vi "console.vi"() -> ()   [LabVIEW 2015]
uses:
  C:/Users/Giuseppe/Downloads/LabLinda_ pakage/index_datatype.ctl
  C:/Users/Giuseppe/Downloads/LabLinda_ pakage/index_cluster.ctl
panel:
  out "Array":cluster{i32}[](array[cluster])
  out "OUTVI REF":string[](array[string])
  out "Key_index":string[](array[string])
  out "Inited ?":bool
  out "IN VI Ref":string[](array[string])
  out "main index":i32
  in  "stop":bool
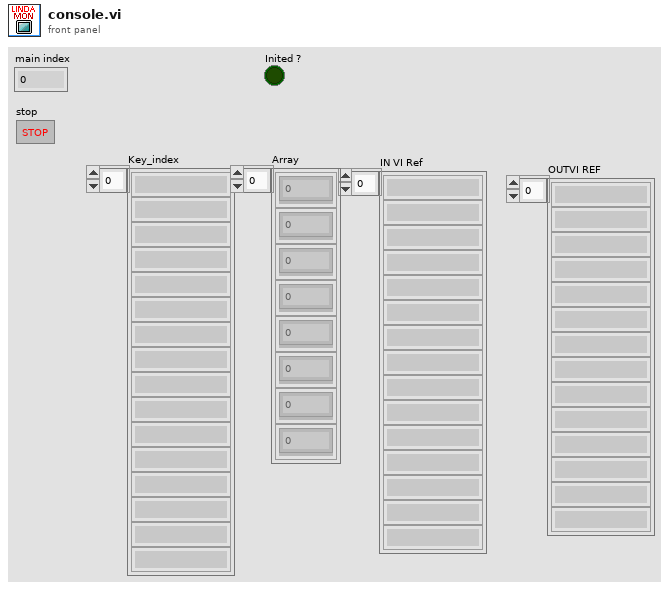
[diagram p1: front panel]
types:
  T1 = typedef "index_datatype.ctl" = T2[]
  T2 = typedef "index_cluster.ctl" = cluster{"Addr":i32[], "out react vi reference":refnum<vi>, "in react vi reference":refnum<vi>, "rd react vi reference":refnum<vi>, "Read_write_var":refnum<vi>}
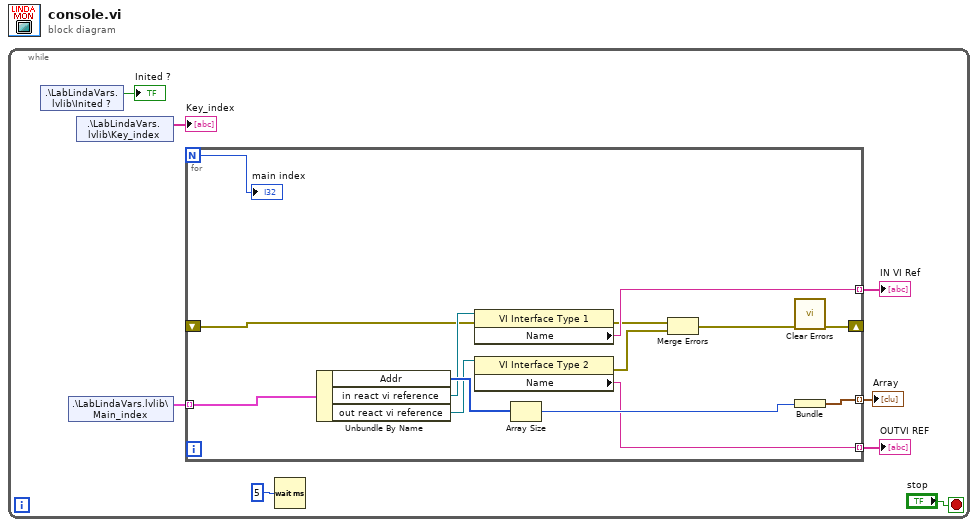
[diagram p0: block diagram]
diagram:
  n1 = while {
    stop <- "stop" stop-if-true
    n2 = shared-variable ".\\LabLindaVars.lvlib\\Inited ?"() -> (→"Inited ?":bool)  [unwired: 1 in, 1 out]
    n3 = shared-variable ".\\LabLindaVars.lvlib\\Main_index"() -> (w5:T1)  [unwired: 1 in, 1 out]
    n4 = shared-variable ".\\LabLindaVars.lvlib\\Key_index"() -> (→"Key_index":string[])  [unwired: 1 in, 1 out]
    n5 = for {
      N -> [w18]
      tunnel: w5 -> [w22] mode=indexing
      tunnel: [w19] -> w1 mode=indexing
      tunnel: [w16] -> w4 mode=indexing
      shift-right: [w14] -> _
      shift-left: _ -> [w15]
      tunnel: [w10] -> w2 mode=indexing
      n6 = Unbundle By Name(w22) -> ("Addr"=w21:i32[], "in react vi reference"=w17:refnum<vi>, "out react vi reference"=w13:refnum<vi>)
      n7 = property class="VI Interface Type 1"(reference=w17, error in=w15) -> (error out=w12:errorcluster, "Name"=w16:string)  [unwired: 1 out]
      n8 = property class="VI Interface Type 2"(reference=w13) -> (error out=w9:errorcluster, "Name"=w10:string)  [unwired: 1 in, 1 out]
      n9 = Array Size(array=w21) -> (size(s)=w20:i32)
      n10 = Merge Errors(w12, w9) -> (w11:errorcluster)
      n11 = call <vilib>:"Clear Errors.vi"("error in (no error)"=w11) -> ("error out"=w14:errorcluster)  [unwired: 5 in, 1 out]
      n12 = Bundle(w20) -> (w19:cluster{i32})  [unwired: 1 in]
      "main index" <- w18
    }
    "IN VI Ref" <- w4
    "OUTVI REF" <- w2
    "Array" <- w1
    n13 = Wait (ms)(milliseconds to wait=u32 5) -> ()  [unwired: 1 out]
  }
